vi "Quadrature BP Noise demo.vi"() -> ()   [LabVIEW 2015]
uses:
  <vilib>/Analysis/NI_AALBase.lvlib
  <vilib>/Analysis/3filter.llb/Filter Passband Type.ctl
  <vilib>/Analysis/3filter.llb/IIR Cascade Filter with I.C. (DBL).vi
  Utility VIs/Math VIs/FFT x(t) to dB,Degrees (1D).vi
  <vilib>/Analysis/1siggen.llb/Ramp Pattern by Samples.vi
  Experiment VIs/Signal Generation VIs/Filter Control/Filter.ctl
panel:
  out "XY Graph":T1(graph)
  out "Waveform Graph":dbl[](graph)
  in  "T (ms)":dbl=1000.0
  in  "Fs (Hz)":dbl=100000.0
  in  "Filter":T2={"CF (kHz)"=5.0, "filter type"=enum."Bandpass", "BW (kHz)"=1.0, "Active"=TRUE, "IIR Filter Cluster"={"filter structure"=enum."IIR 2nd Order", "Reverse Coefficients"=[], "Forward Coefficients"=[]}, "Final Filter State"=[], "Scale Factor"=0.0} {"IIR Filter Cluster"."Forward Coefficients" format="%.4f"; "IIR Filter Cluster"."Reverse Coefficients" format="%.4f"}
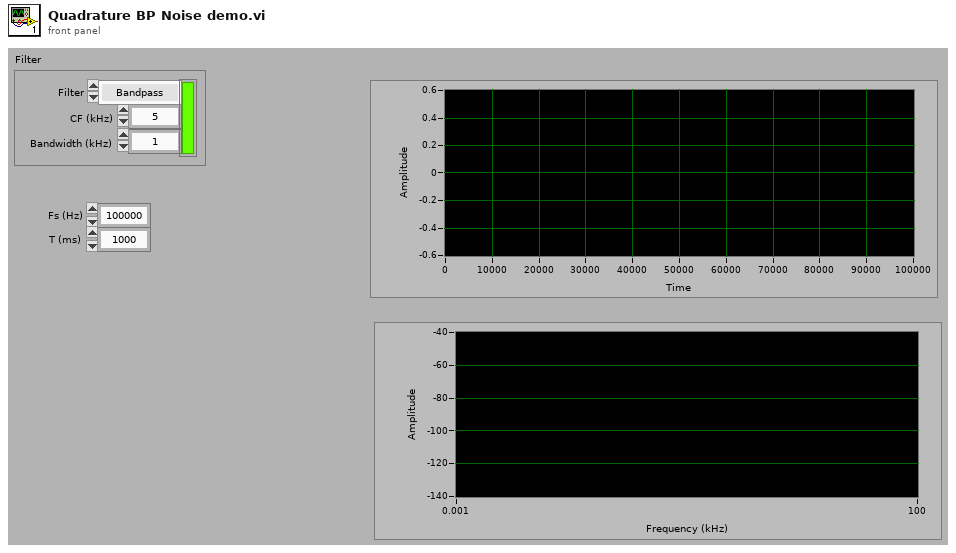
[diagram p1: front panel]
types:
  T1 = cluster{dbl[], "+Freq. Mag of FFT (dB rms)":dbl[]}
  T2 = typedef "Filter.ctl" = cluster{"CF (kHz)":dbl, "filter type":T3, "BW (kHz)":dbl, "Active":bool, "IIR Filter Cluster":cluster{"filter structure":enum32{"IIR 2nd Order", "IIR 4th Order"}, "Reverse Coefficients":dbl[], "Forward Coefficients":dbl[]}, "Final Filter State":dbl[], "Scale Factor":dbl}
  T3 = typedef "NI_AALBase.lvlib/Filter Passband Type.ctl" = enum32{"Lowpass", "Highpass", "Bandpass", "Bandstop"}
  T4 = cluster{"filter structure":enum32{"IIR 2nd Order", "IIR 4th Order"}, "Reverse Coefficients":dbl[], "Forward Coefficients":dbl[]}
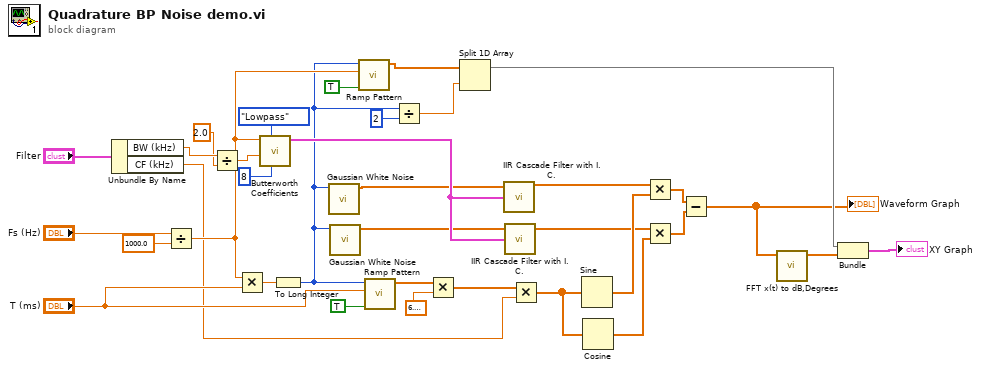
[diagram p0: block diagram]
diagram:
  n1 = Unbundle By Name("Filter") -> ("BW (kHz)"=w4:dbl, "CF (kHz)"=w6:dbl)
  n2 = Divide(x="Fs (Hz)", y=1000.0) -> (x/y=w14:dbl)
  n3 = Divide(x=w4, y=2.0) -> (x/y=w2:dbl)
  n4 = Multiply(x=w14, y="T (ms)") -> (x*y=w31:dbl)
  n5 = call <vilib>:"Butterworth Coefficients.vi"("order"=8, "filter type"=Filter_Passband_Type."Lowpass", "low cutoff freq: fl"=w2, "sampling freq: fs"=w14) -> ("IIR Filter Cluster"=w26:T4)  [unwired: 6 in, 1 out]
  n6 = To Long Integer(number=w31) -> (32bit integer=w12:i32)
  n7 = call <vilib>:"Gaussian White Noise.vi"("samples"=w12) -> ("Gaussian noise pattern"=w24:dbl[])  [unwired: 9 in, 1 out]
  n8 = call <vilib>:"Gaussian White Noise.vi"("samples"=w12) -> ("Gaussian noise pattern"=w25:dbl[])  [unwired: 9 in, 1 out]
  n9 = call-poly <vilib>:"Ramp Pattern.vi"("exclude end?"=TRUE, "end"=w14, "samples"=w12) -> ("Ramp Pattern"=w9:dbl[])  [unwired: 7 in, 1 out]
  n10 = call-poly <vilib>:"Ramp Pattern.vi"("exclude end?"=TRUE, "end"="T (ms)", "samples"=w12) -> ("Ramp Pattern"=w28:dbl[])  [unwired: 7 in, 1 out]
  n11 = Divide(x=w12, y=2) -> (x/y=w10:dbl)
  n12 = Multiply(x=w28, y=6.283185307179586) -> (x*y=w23:dbl[])
  n13 = Split 1D Array(array=w9, index=w10) -> (first subarray=w8:dbl[])  [unwired: 1 out]
  n14 = call-poly <vilib>:"IIR Cascade Filter with I.C..vi"("IIR Filter Cluster"=w26, "X"=w24) -> ("Filtered X"=w16:dbl[])  [unwired: 1 in, 2 out]
  n15 = call-poly <vilib>:"IIR Cascade Filter with I.C..vi"("IIR Filter Cluster"=w26, "X"=w25) -> ("Filtered X"=w20:dbl[])  [unwired: 1 in, 2 out]
  n16 = Multiply(x=w23, y=w6) -> (x*y=w22:dbl[])
  n17 = Sine(x=w22) -> (sin(x)=w21:dbl[])
  n18 = Cosine(x=w22) -> (cos(x)=w19:dbl[])
  n19 = Multiply(x=w16, y=w21) -> (x*y=w18:dbl[])
  n20 = Multiply(x=w20, y=w19) -> (x*y=w17:dbl[])
  n21 = Subtract(x=w18, y=w17) -> (x-y=w3:dbl[])
  "Waveform Graph" <- w3
  n22 = call-poly "FFT x(t) to dB,Degrees.vi"("X"=w3) -> ("+Freq. Mag of FFT (dB rms)"=w13:dbl[])  [unwired: 8 in, 2 out]
  n23 = Bundle(w8, "+Freq. Mag of FFT (dB rms)"=w13) -> (→"XY Graph":T1)  [unwired: 1 in]
